vi "Stop Core.vi"(10 "final error code":i32, 11 "Instr Actor in":refnum<class "Instr Actor.lvclass">) -> (3 "Instr Actor out":refnum<class "Instr Actor.lvclass">)   [LabVIEW 2014, in "Instrument Library.lvlib" / "Instr Actor.lvclass"]
doc: "(<B>Filename</B>: Actor Framework.lvlib:Actor.lvclass:Stop Core.vi)\n\nDefines what the actor does before it stops. Use the <B>final error code</B> input to determine whether the actor shut down in response to an error.\n\nBy default, this method does nothing. A descendant class may override it to define behavior, such as shutting down any processes the actor initiated in its override of the Actor Core method."
uses:
  Instr Actor.lvclass
  Instr Actor.lvclass/Instr Actor.ctl
  reusable/Instrument/Instrument.lvclass/Instrument.ctl
  reusable/Session APIs/Session Log/System Log.lvclass
  reusable/Instrument/Read name.vi
  SuperActor/Ex Nested.lvclass
  <userlib>/_Session Fwk/Session - Root.lvclass
  reusable/Instrument/Instrument.lvclass
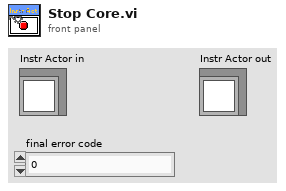
[diagram p1: front panel]
types:
  T1 = typedef "Session - Root.lvclass/Session Handle.ctl" = refnum<data-value>
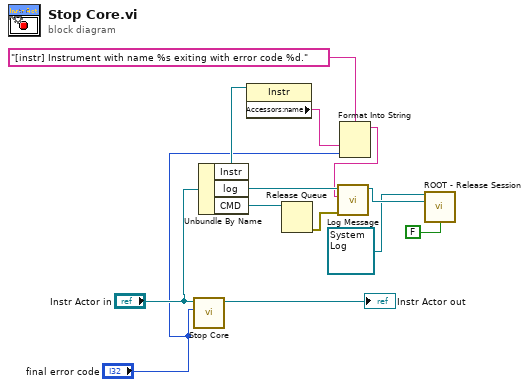
[diagram p0: block diagram]
diagram:
  n1 = call-parent "Stop Core.vi"("final error code"="final error code", "Ex Nested in"="Instr Actor in") -> ("Ex Nested out"=→"Instr Actor out":refnum<class "Instr Actor.lvclass">)  [unwired: 9 in]
  n2 = Unbundle By Name("Instr Actor in") -> ("Instr"=w6:refnum<class "Instrument.lvclass">, "log"=w10:T1, "CMD"=w12:refnum<queue>)
  n3 = property class="Instr"(reference=w6) -> ("Accessors:name"=w4:string)  [unwired: 1 in, 2 out]
  n4 = Release Queue(queue=w12) -> (error out=w7:errorcluster)  [unwired: 2 in, 2 out]
  n5 = Format Into String(format string="[instr] Instrument with name %s exiting with error code %d.", w4, "final error code") -> (resulting string=w2:string)  [unwired: 2 in, 1 out]
  n6 = call "Log Message.vi"("error in"=w7, "MSG In"=w2, "session in"=w10) -> ("session out"=w9:T1)  [unwired: 7 in, 1 out]
  n7 = call <userlib>:"ROOT - Release Session.vi"("OBJ - Session in"=refnum<class "System Log.lvclass"> refnum ("Sys Log"), "Session Handle in"=w9, "force destroy? (F)"=FALSE) -> ()  [unwired: 11 in, 2 out]
